vi "Save Config.vi"(8 "error in (no error)":errorcluster, 11 "Config":T1) -> (0 "error out":errorcluster)   [LabVIEW 2019, in "Config File.lvlib"]
uses:
  Config File.lvlib
  Config Cluster.ctl
  Track Info/Track Info.ctl
  <vilib>/Utility/xml.llb/Write to XML File(string).vi
  Track Info/Track Info.lvlib
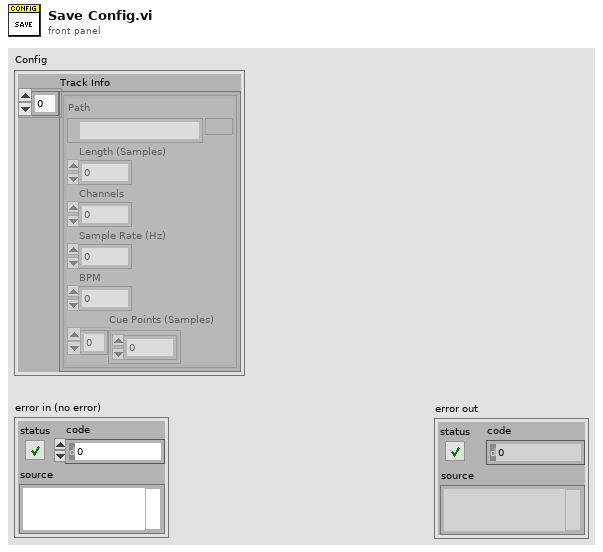
[diagram p1: front panel]
types:
  T1 = typedef "Config File.lvlib/Config Cluster.ctl" = cluster{"Track Info":T2[]}
  T2 = typedef "Track Info.lvlib/Track Info.ctl" = cluster{"Path":path, "Length (Samples)":i32, "Channels":i32, "Sample Rate (Hz)":i32, "BPM":dbl, "Cue Points (Samples)":i32[]}
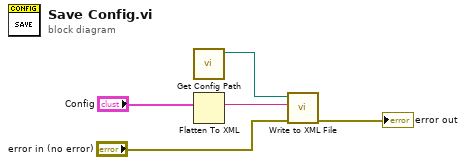
[diagram p0: block diagram]
diagram:
  n1 = call "Get Config Path.vi"() -> ("Config Path"=w3:path)  [unwired: 11 in]
  n2 = Flatten To XML(anything="Config") -> (xml string=w5:string)
  n3 = call-poly <vilib>:"Write to XML File.vi"("error in (no error)"="error in (no error)", "XML Input"=w5, "XML File Path"=w3) -> ("error out"=→"error out":errorcluster)  [unwired: 6 in, 2 out]
